vi "command_move_relative.vi"(8 "error in (no error)":errorcluster, 10 "target  position":refnum<class "SpaceVector.lvclass">, 11 "StageMH110930Scientifica in":refnum<class "StageMH110930Scientifica.lvclass">) -> (0 "error out":errorcluster, 3 "StageMH110930Scientifica out":refnum<class "StageMH110930Scientifica.lvclass">)   [LabVIEW 2010, in "StageMH110930Scientifica.lvclass"]
uses:
  StageMH110930Scientifica.lvclass
  common/classes/SpaceVector/SpaceVector/SpaceVector.lvclass
  common/classes/ErrorController/ErrorController/class_data.vi
  common/classes/ErrorController/ErrorController/ErrorController.lvclass
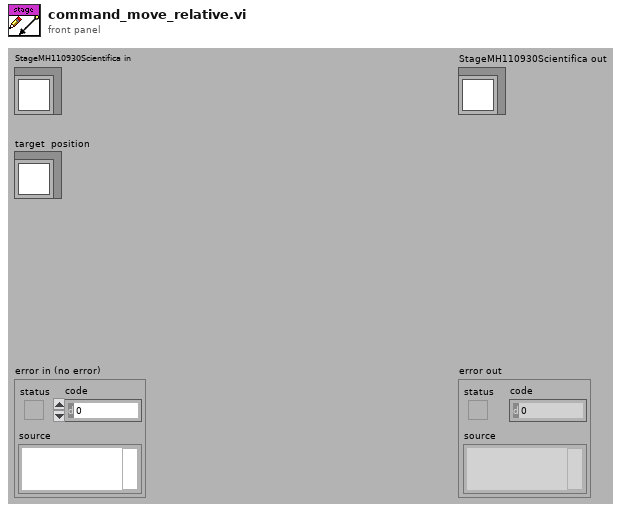
[diagram p1: front panel]
types:
  T1 = typedef "space_vector_array.ctl" = dbl[unit][]
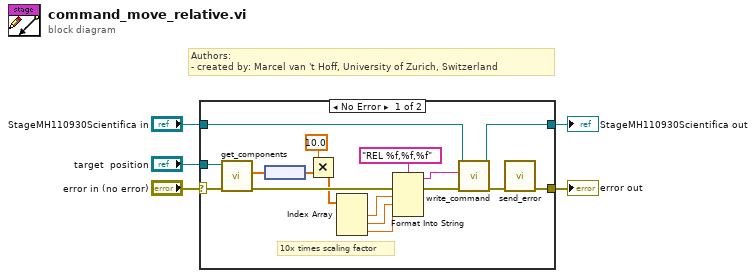
[diagram p0: block diagram]
diagram:
  # "Authors: \n- created by: Marcel van 't Hoff, University of Zurich, Switzerland"
  n1 = case shown="No Error" "error in (no error)" {
    selector: "error in (no error)" -> [w21 w24]
    tunnel: [w10 w24] -> w4
    tunnel: [w11 w23] -> w2
    tunnel: "StageMH110930Scientifica in" -> [w12 w23]
    tunnel: "target  position" -> [w22 _]
    frame No Error {
      # "10x times scaling factor"
      n2 = call "get_components.vi"("error in (no error)"=w21, "SpaceVector in"=w22) -> ("error out"=w14:errorcluster, "x/y/z"=w20:T1)  [unwired: 8 out]
      n3 = node(w20) -> (w9:dbl[])
      n4 = Multiply(x=10.0, y=w9) -> (x*y=w7:dbl[])
      n5 = Index Array(array=w7) -> (element #1=w19:dbl, element #2=w18:dbl, element #3=w17:dbl)  [unwired: 3 in]
      n6 = Format Into String(format string="REL %f,%f,%f", error in=w14, w19, w18, w17) -> (resulting string=w15:string, error out=w13:errorcluster)  [unwired: 1 in]
      n7 = call-dynamic "write_command.vi"("error in (no error)"=w13, "string to write"=w15, "StageMH110930Scientifica in"=w12) -> ("error out"=w8:errorcluster, "StageMH110930Scientifica out"=w11:refnum<class "StageMH110930Scientifica.lvclass">)  [unwired: 5 in, 2 out]
      n8 = call "send_error.vi"("error in (no error)"=w8) -> ("error out"=w10:errorcluster)  [unwired: 10 in]
    }
    frame Error {
    }
  }
  "error out" <- w4
  "StageMH110930Scientifica out" <- w2
